vi "Locate Python Vendors and Versions.vi"(8 "error in (no error)":errorcluster, 11 "object in":refnum<class "JuPyter_Client.lvclass">) -> (0 "error out":errorcluster, 1 "Hives":T1[](array[typedef]), 2 "Python Sub keys":string[](array[string]), 3 "object out":refnum<class "JuPyter_Client.lvclass">)   [LabVIEW 2018, in "JuPyter_Client.lvclass"]
doc: "Use the Windows registry to locate Python Vendors and Versions"
uses:
  JuPyter_Client.lvclass
  <vilib>/registry/registry.llb/Registry RtKey.ctl
  <vilib>/registry/registry.llb/Registry SAM.ctl
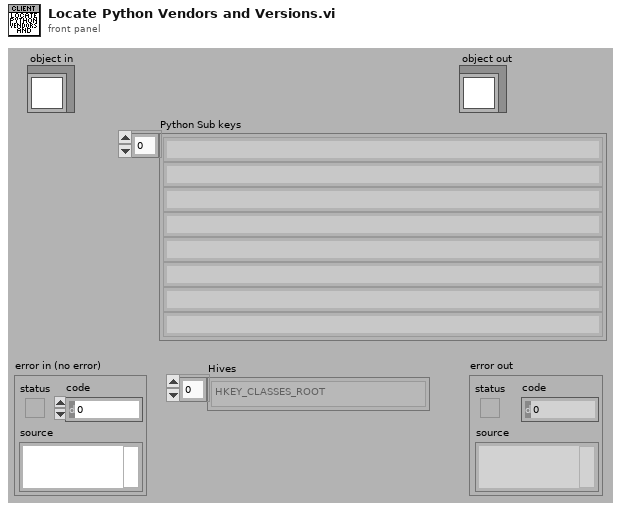
[diagram p1: front panel]
types:
  T1 = typedef "Registry RtKey.ctl" = enum32{"HKEY_CLASSES_ROOT", "HKEY_CURRENT_USER", "HKEY_LOCAL_MACHINE", "HKEY_USERS", "HKEY_PERFORMANCE_DATA", "HKEY_CURRENT_CONFIG", "HKEY_DYN_DATA"}
  T2 = typedef "Registry SAM.ctl" = enum32{"KEY_QUERY_VALUE", "KEY_SET_VALUE", "KEY_CREATE_SUB_KEY", "KEY_ENUMERATE_SUB_KEYS", "KEY_NOTIFY", "KEY_CREATE_LINK", "KEY_READ", "KEY_WRITE", "KEY_ALL_ACCESS", "KEY_READ | KEY_WRITE"}
  T3 = typedef "Registry refnum.ctl" = refnum<k1>
  T4 = cluster{"numSubKeys":i32, "maxSubKeyLen":i32, "maxSubKeyClassLen":i32}
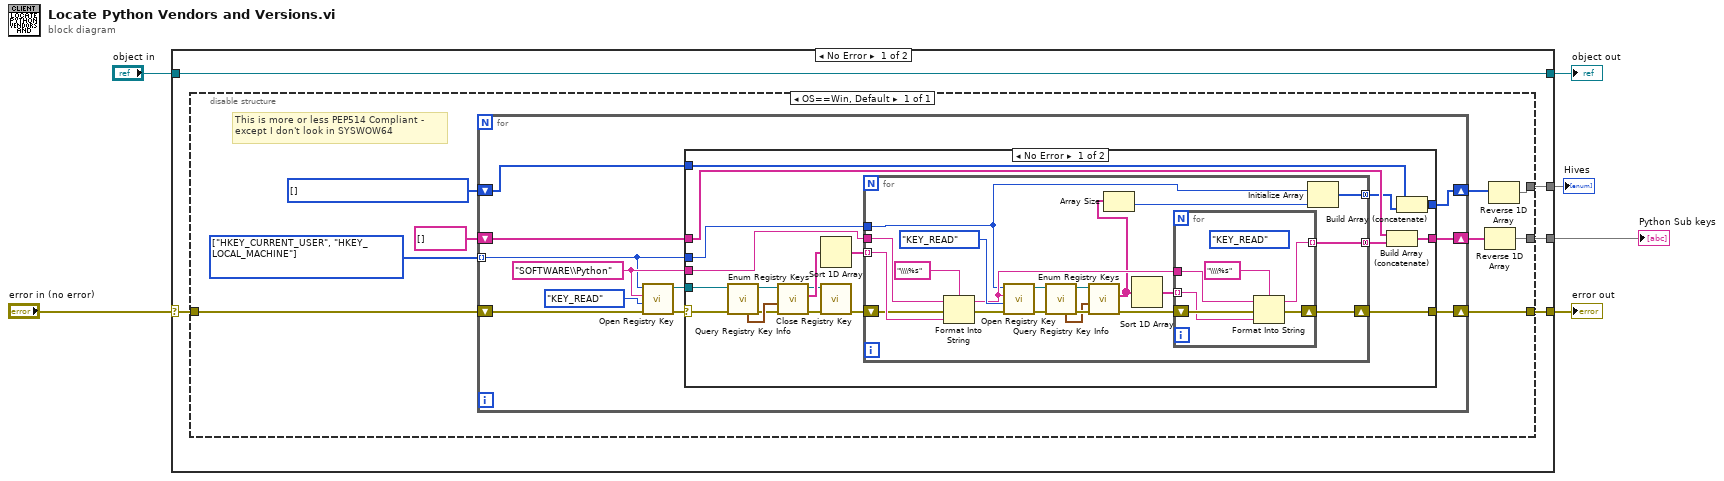
[diagram p0: block diagram]
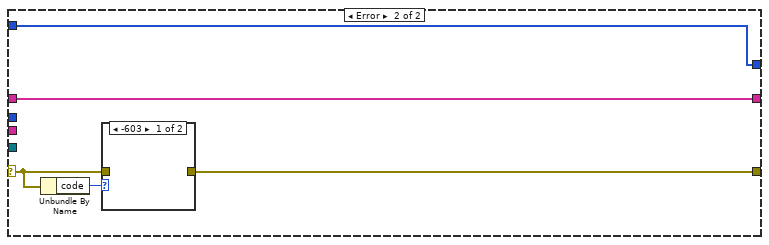
[diagram p2: hidden frame]
diagram:
  n1 = case shown="No Error" "error in (no error)" {
    selector: "error in (no error)" -> [w10 w84]
    tunnel: [w9 w84] -> w5
    tunnel: [w11 w83] -> w3
    tunnel: "object in" -> [w11 w83]
    tunnel: [w8 _] -> w2
    tunnel: [w7 _] -> w1
    frame No Error {
      n2 = disable-structure shown="OS==Win, Default" {
        disable-tunnel: w10 -> [w18]
        disable-tunnel: [w17] -> w9
        disable-tunnel: [w15] -> w8
        disable-tunnel: [w12] -> w7
        frame condition #0 (active) {
          w14 = T1[] [] items=["HKEY_CLASSES_ROOT", "HKEY_CURRENT_USER", "HKEY_LOCAL_MACHINE", "HKEY_USERS", "HKEY_PERFORMANCE_DATA", "HKEY_CURRENT_CONFIG", "HKEY_DYN_DATA"]
          w20 = T1[] [enum."HKEY_CURRENT_USER", enum."HKEY_LOCAL_MACHINE"] items=["HKEY_CLASSES_ROOT", "HKEY_CURRENT_USER", "HKEY_LOCAL_MACHINE", "HKEY_USERS", "HKEY_PERFORMANCE_DATA", "HKEY_CURRENT_CONFIG", "HKEY_DYN_DATA"]
          # "This is more or less PEP514 Compliant - \nexcept I don't look in SYSWOW64"
          n3 = for {
            shift-right: [w27] -> w16
            shift-left: string[] [] -> [w26]
            tunnel: w20 -> [w23] mode=indexing
            shift-right: [w25] -> w17
            shift-left: w18 -> [w24]
            shift-right: [w22] -> w13
            shift-left: w14 -> [w21]
            w28 = "SOFTWARE\\Python" ("subkey")
            n4 = call <vilib>:"Open Registry Key.vi"("error in (no error)"=w24, "security access mask (KEY_READ | KEY_WRITE)"=Registry_SAM."KEY_READ", "subkey"=w28, "root key (HKEY_LOCAL_MACHINE)"=w23) -> ("error out"=w31:errorcluster, "refnum out"=w30:T3)  [unwired: 6 in]
            n5 = case shown="No Error" w31 {
              selector: w31 -> [w49 w78]
              tunnel: w30 -> [w50 _]
              tunnel: w28 -> [w44 _]
              tunnel: w23 -> [w43 _]
              tunnel: [w41 w81] -> w27
              tunnel: w26 -> [w40 w81]
              tunnel: [w35 w79] -> w25
              tunnel: [w33 w77] -> w22
              tunnel: w21 -> [w32 w77]
              frame No Error {
                n6 = call <vilib>:"Query Registry Key Info.vi"("error in (no error)"=w49, "refnum"=w50) -> ("error out"=w46:errorcluster, "refnum out"=w48:T3, "subkey info"=w47:T4)  [unwired: 5 in, 2 out]
                n7 = call <vilib>:"Enum Registry Keys.vi"("error in (no error)"=w46, "subkey info"=w47, "refnum"=w48) -> ("error out"=w39:errorcluster, "subkeys"=w45:string[], "refnum out"=w38:T3)  [unwired: 6 in]
                n8 = Sort 1D Array(array=w45) -> (sorted array=w36:string[])
                n9 = call <vilib>:"Close Registry Key.vi"("error in (no error)"=w39, "refnum"=w38) -> ("error out"=w37:errorcluster)  [unwired: 5 in]
                n10 = for {
                  tunnel: w36 -> [w68] mode=indexing
                  tunnel: w44 -> [w70]
                  tunnel: w43 -> [w53]
                  shift-right: [w59] -> w35
                  shift-left: w37 -> [w66]
                  tunnel: [w58] -> w42 mode=concatenating
                  tunnel: [w52] -> w34 mode=concatenating
                  n11 = Format Into String(format string="\\\\%s", initial string=w70, error in=w66, w68) -> (resulting string=w61:string, error out=w67:errorcluster)
                  n12 = call <vilib>:"Open Registry Key.vi"("error in (no error)"=w67, "security access mask (KEY_READ | KEY_WRITE)"=Registry_SAM."KEY_READ", "subkey"=w61, "root key (HKEY_LOCAL_MACHINE)"=w53) -> ("error out"=w55:errorcluster, "refnum out"=w56:T3)  [unwired: 6 in]
                  n13 = call <vilib>:"Query Registry Key Info.vi"("error in (no error)"=w55, "refnum"=w56) -> ("error out"=w65:errorcluster, "refnum out"=w63:T3, "subkey info"=w64:T4)  [unwired: 5 in, 2 out]
                  n14 = call <vilib>:"Enum Registry Keys.vi"("error in (no error)"=w65, "subkey info"=w64, "refnum"=w63) -> ("error out"=w60:errorcluster, "subkeys"=w54:string[])  [unwired: 6 in, 1 out]
                  n15 = Array Size(array=w54) -> (size(s)=w51:i32)
                  n16 = Sort 1D Array(array=w54) -> (sorted array=w57:string[])
                  n17 = for {
                    tunnel: w61 -> [w75]
                    tunnel: w57 -> [w71] mode=indexing
                    shift-right: [w73] -> w59
                    shift-left: w60 -> [w74]
                    tunnel: [w72] -> w58 mode=indexing
                    (unwired) Registry_SAM."KEY_READ" ("security access mask (KEY_READ | KEY_WRITE)")
                    n18 = Format Into String(format string="\\\\%s", initial string=w75, error in=w74, w71) -> (resulting string=w72:string, error out=w73:errorcluster)
                  }
                  n19 = Initialize Array(w53, w51) -> (w52:T1[])
                }
                n20 = Build Array (concatenate)(w40, w42) -> (w41:string[])
                n21 = Build Array (concatenate)(w32, w34) -> (w33:T1[])
              }
              frame Error {
                n22 = Unbundle By Name(w78) -> ("code"=w80:i32)
                n23 = case shown="-603" w80 {
                  tunnel: [_ w82] -> w79
                  tunnel: w78 -> [_ w82]
                  frame -603 {
                  }
                  frame 1, Default {
                  }
                }
              }
            }
          }
          n24 = Reverse 1D Array(array=w16) -> (reversed array=w15:string[])
          n25 = Reverse 1D Array(array=w13) -> (reversed array=w12:T1[])
        }
      }
    }
    frame Error {
    }
  }
  "error out" <- w5
  "object out" <- w3
  "Python Sub keys" <- w2
  "Hives" <- w1
